vi "Ju move.vi"(1 "Color":i32, 2 "Array Position":cluster{"Row":i32, "Column":i32}, 3 "Chess Array":i32[][](array[numeric])=[[140, 130, 120, 110, 100, 111, 121, 131, 141], [-1, -1, -1, -1, -1, -1, -1, -1, -1], [-1, 150, -1, -1, -1, -1, -1, 151, -1], [160, -1, 161, -1, 162, -1, 163, -1, 164], [-1, -1, -1, -1, -1, -1, -1, -1, -1], [-1, -1, -1, -1, -1, -1, -1, -1, -1], [260, -1, 261, -1, 262, -1, 263, -1, 264], [-1, 250, -1, -1, -1, -1, -1, 251, -1], [-1, -1, -1, -1, -1, -1, -1, -1, -1], [240, 230, 220, 210, 200, 211, 221, 231, 241]]) -> (0 "Ju move":cluster{"Row":i32, i32}[](array[cluster]))   [LabVIEW 2009]
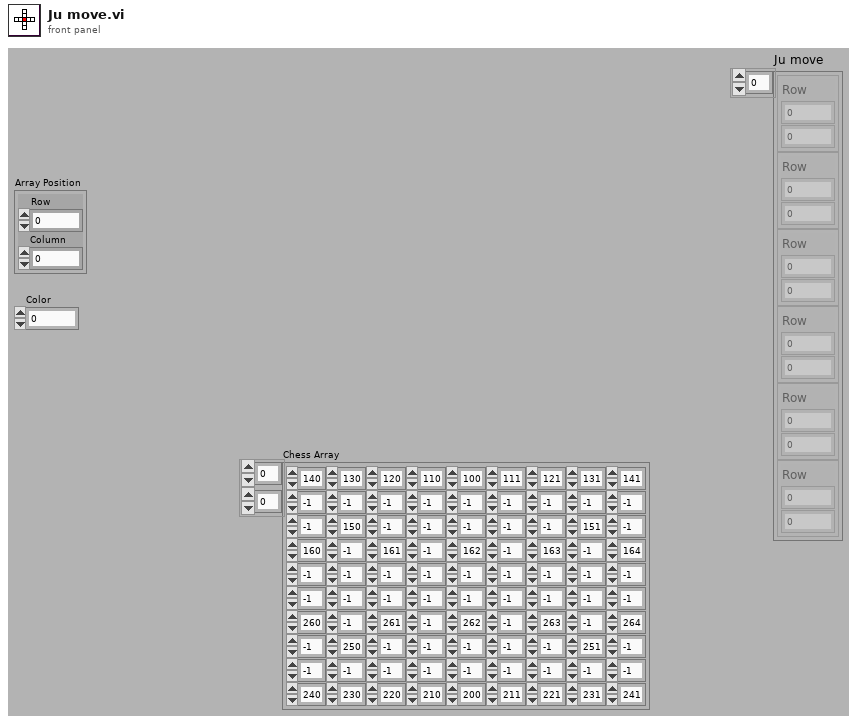
[diagram p1: front panel]
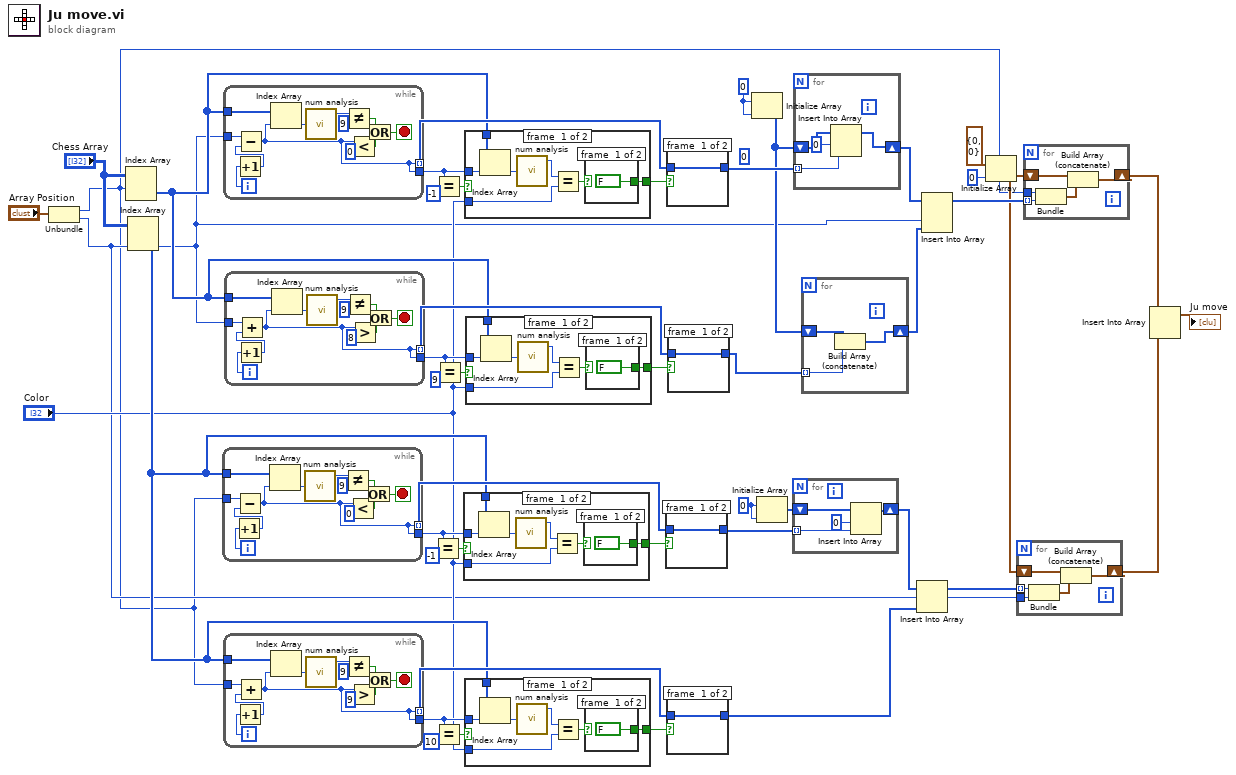
[diagram p0: block diagram]
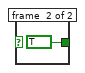
[diagram p2: hidden frame]
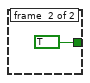
[diagram p3: hidden frame]
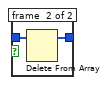
[diagram p4: hidden frame]
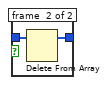
[diagram p5: hidden frame]
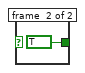
[diagram p6: hidden frame]
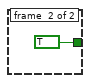
[diagram p7: hidden frame]
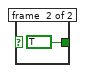
[diagram p8: hidden frame]
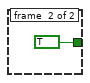
[diagram p9: hidden frame]
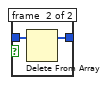
[diagram p10: hidden frame]
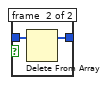
[diagram p11: hidden frame]
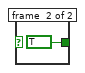
[diagram p12: hidden frame]
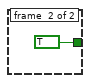
[diagram p13: hidden frame]
diagram:
  w14 = 0
  (unwired) 0
  w25 = 0 ("Element Data")
  n1 = Unbundle("Array Position") -> ("Row"=w2:i32, "Column"=w5:i32)
  n2 = Index Array(array="Chess Array", index (row)=w2) -> (element=w35:i32[])  [unwired: 1 in]
  n3 = Index Array(array="Chess Array", index (col)=w5) -> (element=w18:i32[])  [unwired: 1 in]
  n4 = while {
    tunnel: w18 -> [w58]
    tunnel: w2 -> [w50]
    tunnel: [w47] -> w19 mode=indexing
    tunnel: [w47] -> w22
    i -> [w49]
    stop <- w53 stop-if-true
    n5 = Increment(x=w49) -> (x+1=w48:i32)
    n6 = Subtract(x=w50, y=w48) -> (x-y=w47:i32)
    n7 = Index Array(array=w58, index=w47) -> (element=w56:i32)
    n8 = call "num analysis.vi"("x"=w56) -> ("Color"=w52:i32)  [unwired: 2 out]
    n9 = Not Equal?(x=w52, y=9) -> (x != y?=w51:bool)
    n10 = Less?(x=w47, y=0) -> (x < y?=w54:bool)
    n11 = Or(x=w51, y=w54) -> (x .or. y?=w53:bool)
  }
  n12 = while {
    tunnel: w35 -> [w70]
    tunnel: w5 -> [w62]
    tunnel: [w59] -> w45 mode=indexing
    tunnel: [w59] -> w42
    i -> [w61]
    stop <- w65 stop-if-true
    n13 = Increment(x=w61) -> (x+1=w60:i32)
    n14 = Subtract(x=w62, y=w60) -> (x-y=w59:i32)
    n15 = Index Array(array=w70, index=w59) -> (element=w68:i32)
    n16 = call "num analysis.vi"("x"=w68) -> ("Color"=w64:i32)  [unwired: 2 out]
    n17 = Not Equal?(x=w64, y=9) -> (x != y?=w63:bool)
    n18 = Less?(x=w59, y=0) -> (x < y?=w66:bool)
    n19 = Or(x=w63, y=w66) -> (x .or. y?=w65:bool)
  }
  n20 = while {
    tunnel: w18 -> [w82]
    tunnel: w2 -> [w74]
    tunnel: [w71] -> w30 mode=indexing
    tunnel: [w71] -> w27
    i -> [w73]
    stop <- w77 stop-if-true
    n21 = Increment(x=w73) -> (x+1=w72:i32)
    n22 = Add(x=w74, y=w72) -> (x+y=w71:i32)
    n23 = Index Array(array=w82, index=w71) -> (element=w80:i32)
    n24 = call "num analysis.vi"("x"=w80) -> ("Color"=w76:i32)  [unwired: 2 out]
    n25 = Not Equal?(x=w76, y=9) -> (x != y?=w75:bool)
    n26 = Greater?(x=w71, y=9) -> (0:w78:bool)
    n27 = Or(x=w75, y=w78) -> (x .or. y?=w77:bool)
  }
  n28 = while {
    tunnel: w35 -> [w94]
    tunnel: w5 -> [w86]
    tunnel: [w83] -> w36 mode=indexing
    tunnel: [w83] -> w39
    i -> [w85]
    stop <- w89 stop-if-true
    n29 = Increment(x=w85) -> (x+1=w84:i32)
    n30 = Add(x=w86, y=w84) -> (x+y=w83:i32)
    n31 = Index Array(array=w94, index=w83) -> (element=w92:i32)
    n32 = call "num analysis.vi"("x"=w92) -> ("Color"=w88:i32)  [unwired: 2 out]
    n33 = Not Equal?(x=w88, y=9) -> (x != y?=w87:bool)
    n34 = Greater?(x=w83, y=8) -> (0:w90:bool)
    n35 = Or(x=w87, y=w90) -> (x .or. y?=w89:bool)
  }
  n36 = Equal?(x=w22, y=-1) -> (x = y?=w21:bool)
  n37 = Equal?(x=w42, y=-1) -> (x = y?=w43:bool)
  n38 = Equal?(x=w27, y=10) -> (x = y?=w28:bool)
  n39 = Equal?(x=w39, y=9) -> (x = y?=w38:bool)
  n40 = case shown="False" w21 {
    tunnel: w18 -> [w101 _]
    tunnel: w22 -> [w100 _]
    tunnel: "Color" -> [w97 _]
    tunnel: [w95 TRUE] -> w23
    frame #0 {
      n41 = Index Array(array=w101, index=w100) -> (element=w99:i32)
      n42 = call "num analysis.vi"("x"=w99) -> ("Color"=w98:i32)  [unwired: 2 out]
      n43 = Equal?(x=w98, y=w97) -> (x = y?=w96:bool)
      n44 = case shown="False" w96 {
        tunnel: [FALSE TRUE] -> w95
        frame #0 {
        }
        frame #1 {
        }
      }
    }
    frame #1 {
    }
  }
  n45 = case shown="False" w43 {
    tunnel: w35 -> [w111 _]
    tunnel: w42 -> [w110 _]
    tunnel: "Color" -> [w107 _]
    tunnel: [w105 TRUE] -> w41
    frame #0 {
      n46 = Index Array(array=w111, index=w110) -> (element=w109:i32)
      n47 = call "num analysis.vi"("x"=w109) -> ("Color"=w108:i32)  [unwired: 2 out]
      n48 = Equal?(x=w108, y=w107) -> (x = y?=w106:bool)
      n49 = case shown="False" w106 {
        tunnel: [FALSE TRUE] -> w105
        frame #0 {
        }
        frame #1 {
        }
      }
    }
    frame #1 {
    }
  }
  n50 = case shown="False" w28 {
    tunnel: w18 -> [w121 _]
    tunnel: w27 -> [w120 _]
    tunnel: "Color" -> [w117 _]
    tunnel: [w115 TRUE] -> w26
    frame #0 {
      n51 = Index Array(array=w121, index=w120) -> (element=w119:i32)
      n52 = call "num analysis.vi"("x"=w119) -> ("Color"=w118:i32)  [unwired: 2 out]
      n53 = Equal?(x=w118, y=w117) -> (x = y?=w116:bool)
      n54 = case shown="False" w116 {
        tunnel: [FALSE TRUE] -> w115
        frame #0 {
        }
        frame #1 {
        }
      }
    }
    frame #1 {
    }
  }
  n55 = case shown="False" w38 {
    tunnel: w35 -> [w131 _]
    tunnel: w39 -> [w130 _]
    tunnel: "Color" -> [w127 _]
    tunnel: [w125 TRUE] -> w40
    frame #0 {
      n56 = Index Array(array=w131, index=w130) -> (element=w129:i32)
      n57 = call "num analysis.vi"("x"=w129) -> ("Color"=w128:i32)  [unwired: 2 out]
      n58 = Equal?(x=w128, y=w127) -> (x = y?=w126:bool)
      n59 = case shown="False" w126 {
        tunnel: [FALSE TRUE] -> w125
        frame #0 {
        }
        frame #1 {
        }
      }
    }
    frame #1 {
    }
  }
  n60 = case shown="True" w23 {
    tunnel: w19 -> [w135 w137]
    tunnel: [w135 w136] -> w32
    frame #0 {
    }
    frame #1 {
      n61 = Delete From Array(array=w137) -> (array with subset deleted=w136:i32[])  [unwired: 2 in, 1 out]
    }
  }
  n62 = case shown="True" w41 {
    tunnel: w45 -> [w138 w140]
    tunnel: [w138 w139] -> w33
    frame #0 {
    }
    frame #1 {
      n63 = Delete From Array(array=w140) -> (array with subset deleted=w139:i32[])  [unwired: 2 in, 1 out]
    }
  }
  n64 = case shown="True" w26 {
    tunnel: w30 -> [w141 w143]
    tunnel: [w141 w142] -> w1
    frame #0 {
    }
    frame #1 {
      n65 = Delete From Array(array=w143) -> (array with subset deleted=w142:i32[])  [unwired: 2 in, 1 out]
    }
  }
  n66 = case shown="True" w40 {
    tunnel: w36 -> [w144 w146]
    tunnel: [w144 w145] -> w15
    frame #0 {
    }
    frame #1 {
      n67 = Delete From Array(array=w146) -> (array with subset deleted=w145:i32[])  [unwired: 2 in, 1 out]
    }
  }
  n68 = Initialize Array(w14, w14) -> (w13:i32[])
  n69 = Initialize Array(w25, w25) -> (w24:i32[])
  n70 = for {
    shift-right: [w148] -> w31
    shift-left: w24 -> [w149]
    tunnel: w32 -> [w147] mode=indexing
    n71 = Insert Into Array(array=w149, index=0 ("Index"), new element=w147) -> (w148:i32[])
  }
  n72 = for {
    shift-right: [w153] -> w34
    shift-left: w13 -> [w154]
    tunnel: w33 -> [w152] mode=indexing
    n73 = Insert Into Array(array=w154, index=0 ("Index"), new element=w152) -> (w153:i32[])
  }
  n74 = for {
    tunnel: w15 -> [w156] mode=indexing
    shift-right: [w155] -> w12
    shift-left: w13 -> [w157]
    n75 = Build Array (concatenate)(w157, w156) -> (w155:i32[])
  }
  n76 = Insert Into Array(array=w31, new element=w1) -> (w6:i32[])  [unwired: 1 in]
  n77 = Insert Into Array(array=w34, new element #1=w5, new element #2=w12) -> (w11:i32[])  [unwired: 1 in]
  n78 = Initialize Array(cluster{"Row":i32, i32} {"Row"=0, 0} ("Output Cluster"), 0 ("Dimension Size")) -> (w8:cluster{"Row":i32, i32}[])
  n79 = for {
    shift-right: [w160] -> w4
    shift-left: w8 -> [w161]
    tunnel: w6 -> [w159] mode=indexing
    tunnel: w5 -> [w158]
    n80 = Bundle("Element Data"=w159, "Column"=w158) -> (w162:cluster{"Element Data":i32, "Column":i32})  [unwired: 1 out]
    n81 = Build Array (concatenate)(w161, w162) -> (w160:cluster{"Element Data":i32, "Column":i32}[])
  }
  n82 = for {
    tunnel: w2 -> [w167]
    tunnel: w11 -> [w166] mode=indexing
    shift-right: [w163] -> w7
    shift-left: w8 -> [w164]
    n83 = Bundle("Row"=w167, w166) -> (w165:cluster{"Row":i32, i32})  [unwired: 1 out]
    n84 = Build Array (concatenate)(w164, w165) -> (w163:cluster{"Row":i32, i32}[])
  }
  n85 = Insert Into Array(array=w7, new element=w4) -> (→"Ju move":cluster{"Row":i32, i32}[])  [unwired: 1 in]
